vi "Simple Waveform Creator (Debug).vi"() -> ()   [LabVIEW 2021]
uses:
  <vilib>/express/express signal manip/GetorSetDDTAttributes/Get DDT Attributes/Get DDT Properties.xnode
  <vilib>/express/express shared/transition.llb/Dynamic To Waveform Array.vi
panel:
  out "Dt":dbl[](array[numeric])
  out "Array of Waveforms":waveform(dbl)[](array[waveform])=[{"t0"=timestamp(0 s since 1904-01-01), "dt"=0.001, "Y"=array[999 elements], "attributes"=variant("NI_ChannelName"=variant(string "Sine (Resampled)"), "NI_ExpIsRelativeTime"=variant(bool TRUE), "NI_ExpStartTimeStamp"=variant(timestamp timestamp(3848030461.1611934 s since 1904-01-01)), "NI_ExpTimeStamp"=variant(timestamp timestamp(3848030461.1611934 s since 1904-01-01)), "NI_ExpXDimension"=variant(string "t"), "NI_OriginalChannelName"=variant(string "Sine"))}, {"t0"=timestamp(0 s since 1904-01-01), "dt"=0.001, "Y"=array[915 elements], "attributes"=variant("NI_ChannelName"=variant(string "Triangle (Resampled)"), "NI_ExpIsRelativeTime"=variant(bool TRUE), "NI_ExpStartTimeStamp"=variant(timestamp timestamp(3848030461.160188 s since 1904-01-01)), "NI_ExpTimeStamp"=variant(timestamp timestamp(3848030461.160188 s since 1904-01-01)), "NI_ExpXDimension"=variant(string "t"), "NI_OriginalChannelName"=variant(string "Triangle"))}]
  out "Waveforms Graph":dynamicdata(graph) caption="Resampled Signals 2"
  out "Names":string[](array[string])
  out "Duration":dbl[](array[numeric])
  out "Size":i32[](array[numeric])
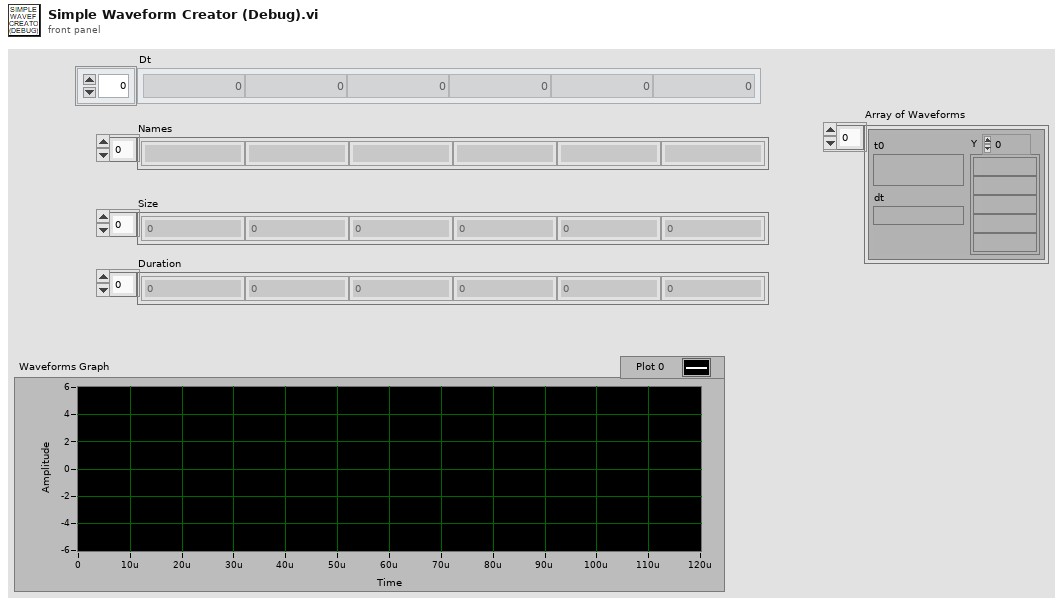
[diagram p1: front panel]
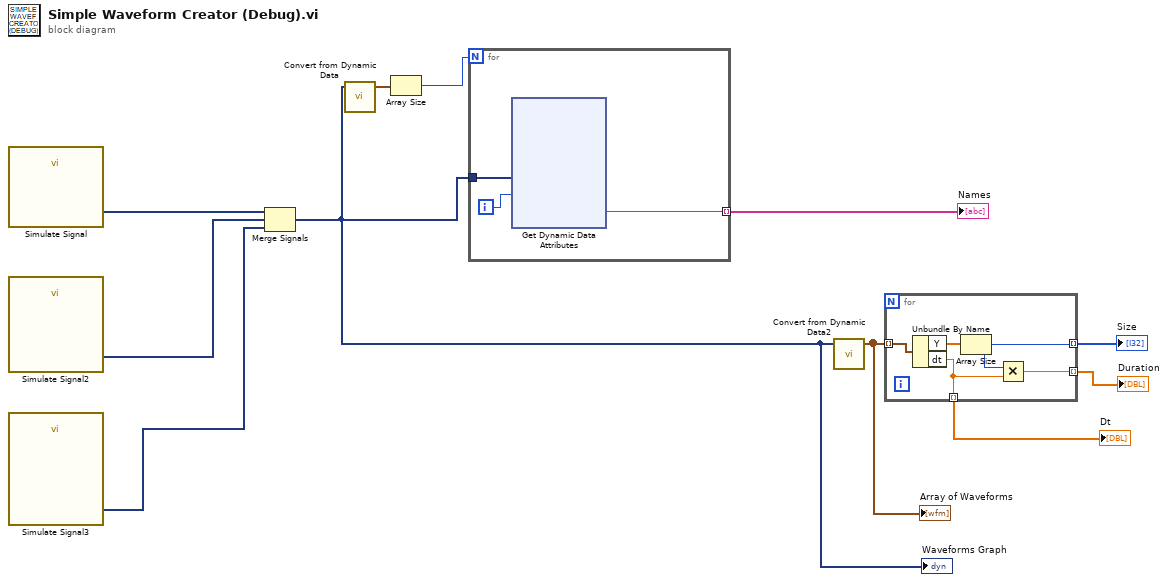
[diagram p0: block diagram]
diagram:
  n1 = call "Simulate Signal"() -> ("DcOff10us"=w9:dynamicdata)  [unwired: 14 in, 1 out]
  n2 = call "Simulate Signal2"() -> ("DcOn120us"=w8:dynamicdata)  [unwired: 14 in, 1 out]
  n3 = call "Simulate Signal3"() -> ("Sine1kHz100us"=w6:dynamicdata)  [unwired: 14 in, 1 out]
  n4 = Merge Signals(w9, w8, w6) -> (w1:dynamicdata)
  "Waveforms Graph" <- w1
  n5 = call "Convert from Dynamic Data"("Dynamic Data Type"=w1) -> ("Array of Waveform"=w4:waveform(dbl)[])  [unwired: 3 in]
  n6 = Array Size(array=w4) -> (size(s)=w2:i32)
  n7 = for {
    N: w2 -> [_]
    tunnel: w1 -> [w14]
    tunnel: [w13] -> w3 mode=indexing
    i -> [w12]
    n8 = xnode "Get Dynamic Data Attributes"("Signals In"=w14, "Signal Index"=w12) -> ("Signal Name"=w13:string)  [unwired: 1 in, 2 out]
  }
  "Names" <- w3
  n9 = call "Convert from Dynamic Data2"("Dynamic Data Type"=w1) -> ("Array of Waveform"=w7:waveform(dbl)[])  [unwired: 3 in]
  "Array of Waveforms" <- w7
  n10 = for {
    tunnel: w7 -> [w28] mode=indexing
    tunnel: [w26] -> w10 mode=indexing
    tunnel: [w25] -> w11 mode=indexing
    tunnel: [w24] -> w5 mode=indexing
    n11 = Unbundle By Name(w28) -> ("Y"=w27:dbl[], "dt"=w24:dbl)
    n12 = Array Size(array=w27) -> (size(s)=w25:i32)
    n13 = Multiply(x=w25, y=w24) -> (x*y=w26:dbl)
  }
  "Size" <- w11
  "Duration" <- w10
  "Dt" <- w5
